vi "setEndRampEvent.vi"(8 "error in (no error)":errorcluster, 10 "EndScriptEvent":refnum<class "ScriptEvent.lvclass">, 11 "RampAction in":refnum<class "RampAction.lvclass">) -> (0 "error out":errorcluster, 3 "RampAction out":refnum<class "RampAction.lvclass">)   [LabVIEW 2009, in "Views.lvlib" / "ScriptEditor.lvlib" / "RampAction.lvclass"]
uses:
  RampAction.lvclass
  Tools/Scripting/ScriptingEvent/ScriptEvent.lvclass
  Tools/Scripting/ScriptingEvent/ScriptEvents/Ramp/RampEvent/RampEvent.lvclass
  ActionPanel.lvclass
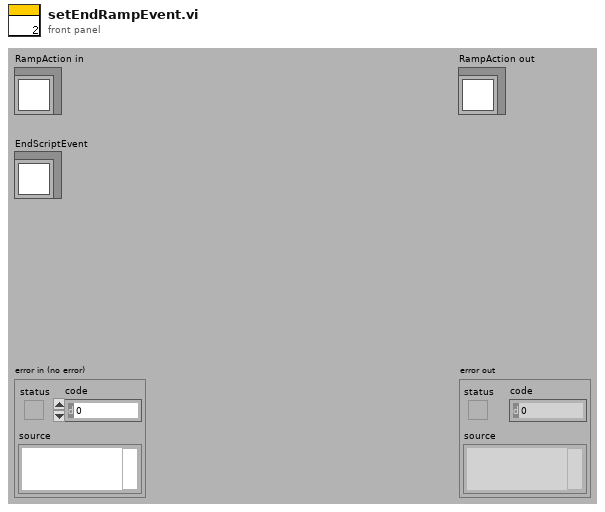
[diagram p1: front panel]
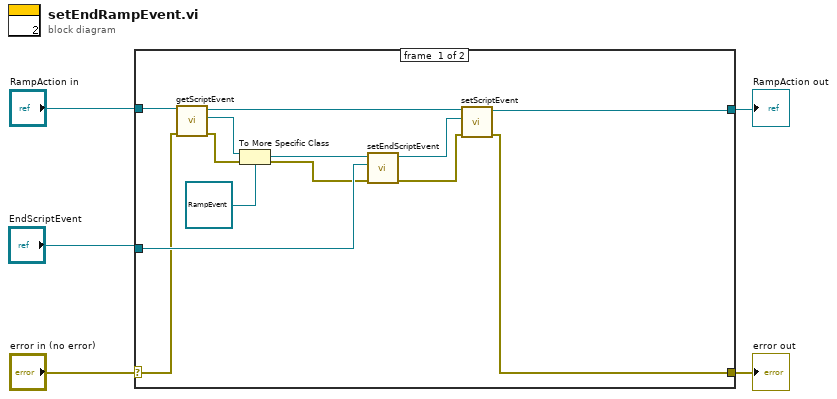
[diagram p0: block diagram]
diagram:
  n1 = case shown="No Error" "error in (no error)" {
    selector: "error in (no error)" -> [w7 w20]
    tunnel: [w6 w20] -> w4
    tunnel: "RampAction in" -> [w18 w19]
    tunnel: [w10 w19] -> w2
    tunnel: "EndScriptEvent" -> [w13 _]
    frame #0 {
      n2 = call "getScriptEvent.vi"("error in (no error)"=w7, "ActionPanel.lvclass in"=w18) -> ("error out"=w15:errorcluster, "ScriptEvent.lvclass"=w17:refnum<class "ScriptEvent.lvclass">, "ActionPanel.lvclass out"=w11:refnum<class "RampAction.lvclass">)  [unwired: 7 in]
      n3 = To More Specific Class(target class=refnum<class "RampEvent.lvclass"> refnum ("Tools.lvlib:Scripting.lvlib:RampEvent.lvclass"), reference=w17, error in=w15) -> (specific class reference=w14:refnum<class "RampEvent.lvclass">, error out=w12:errorcluster)
      n4 = call "setEndScriptEvent.vi"("error in (no error)"=w12, "endScriptEvent.lvclass"=w13, "RampEvent.lvclass in"=w14) -> ("error out"=w8:errorcluster, "RampEvent.lvclass out"=w9:refnum<class "RampEvent.lvclass">)  [unwired: 7 in]
      n5 = call "setScriptEvent.vi"("error in (no error)"=w8, "ScriptEvent.lvclass"=w9, "ActionPanel.lvclass in"=w11) -> ("error out"=w6:errorcluster, "ActionPanel.lvclass out"=w10:refnum<class "RampAction.lvclass">)  [unwired: 7 in]
    }
    frame #1 {
    }
  }
  "error out" <- w4
  "RampAction out" <- w2
